vi "M100Utilization1.vi"() -> ()   [LabVIEW 2012]
uses:
  <vilib>/Utility/NIReport.llb/NI_report.lvclass
  <vilib>/addons/database/Connection.llb/DB Tools Open Connec (Path).vi
  <vilib>/addons/database/Connection.llb/Conn Execute.vi
  <vilib>/addons/database/Recordset.llb/Rec Fetch Recordset Data (R).vi
  <vilib>/addons/database/Recordset.llb/Rec Destroy - Connection.vi
  <vilib>/Utility/NIReport.llb/Append Text Table to Report (wrap).vi
  <vilib>/addons/database/_DB Variant To Data/Database Variant To Data.xnode
  <vilib>/addons/database/NI_Database_API.lvlib
  <vilib>/Utility/NIReport.llb/Excel/NI_Excel.lvclass
  <vilib>/addons/_office/NI_ReportGenerationToolkit.lvlib
  <vilib>/Utility/SMTP/NI_SMTPEmail.lvlib
panel:
  in  "Report Template":path=path "O:/Monitor/Report/M100DailyUtilization1.xls"
  out "error out 2":errorcluster
  in  "Table Control":string[][](table)
  out "error out":errorcluster
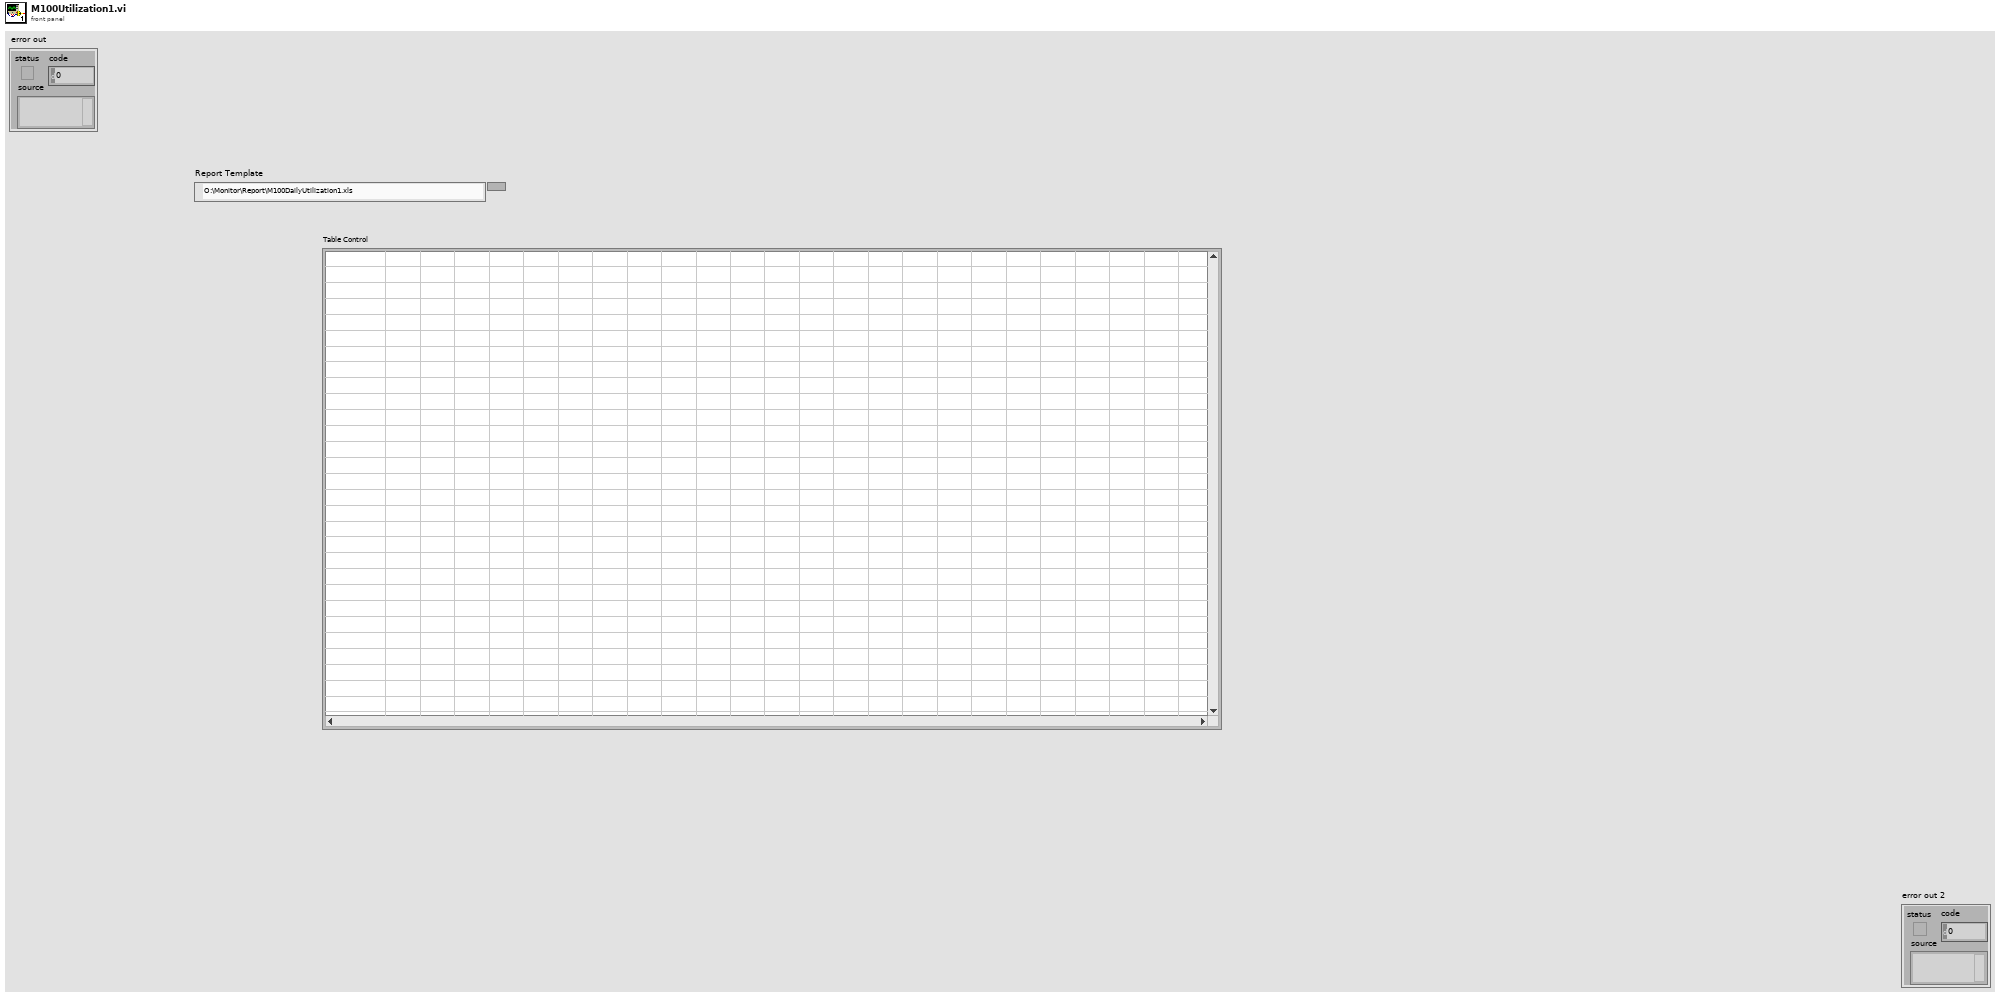
[diagram p1: front panel]
types:
  T1 = typedef "NI_Database_API.lvlib/Conn ObjectReference.ctl" = refnum<k1>
  T2 = typedef "NI_Database_API.lvlib/Rec ObjectReference.ctl" = refnum<k1>
  T3 = enum16{"Standard Report", "HTML", "Word", "Excel"}
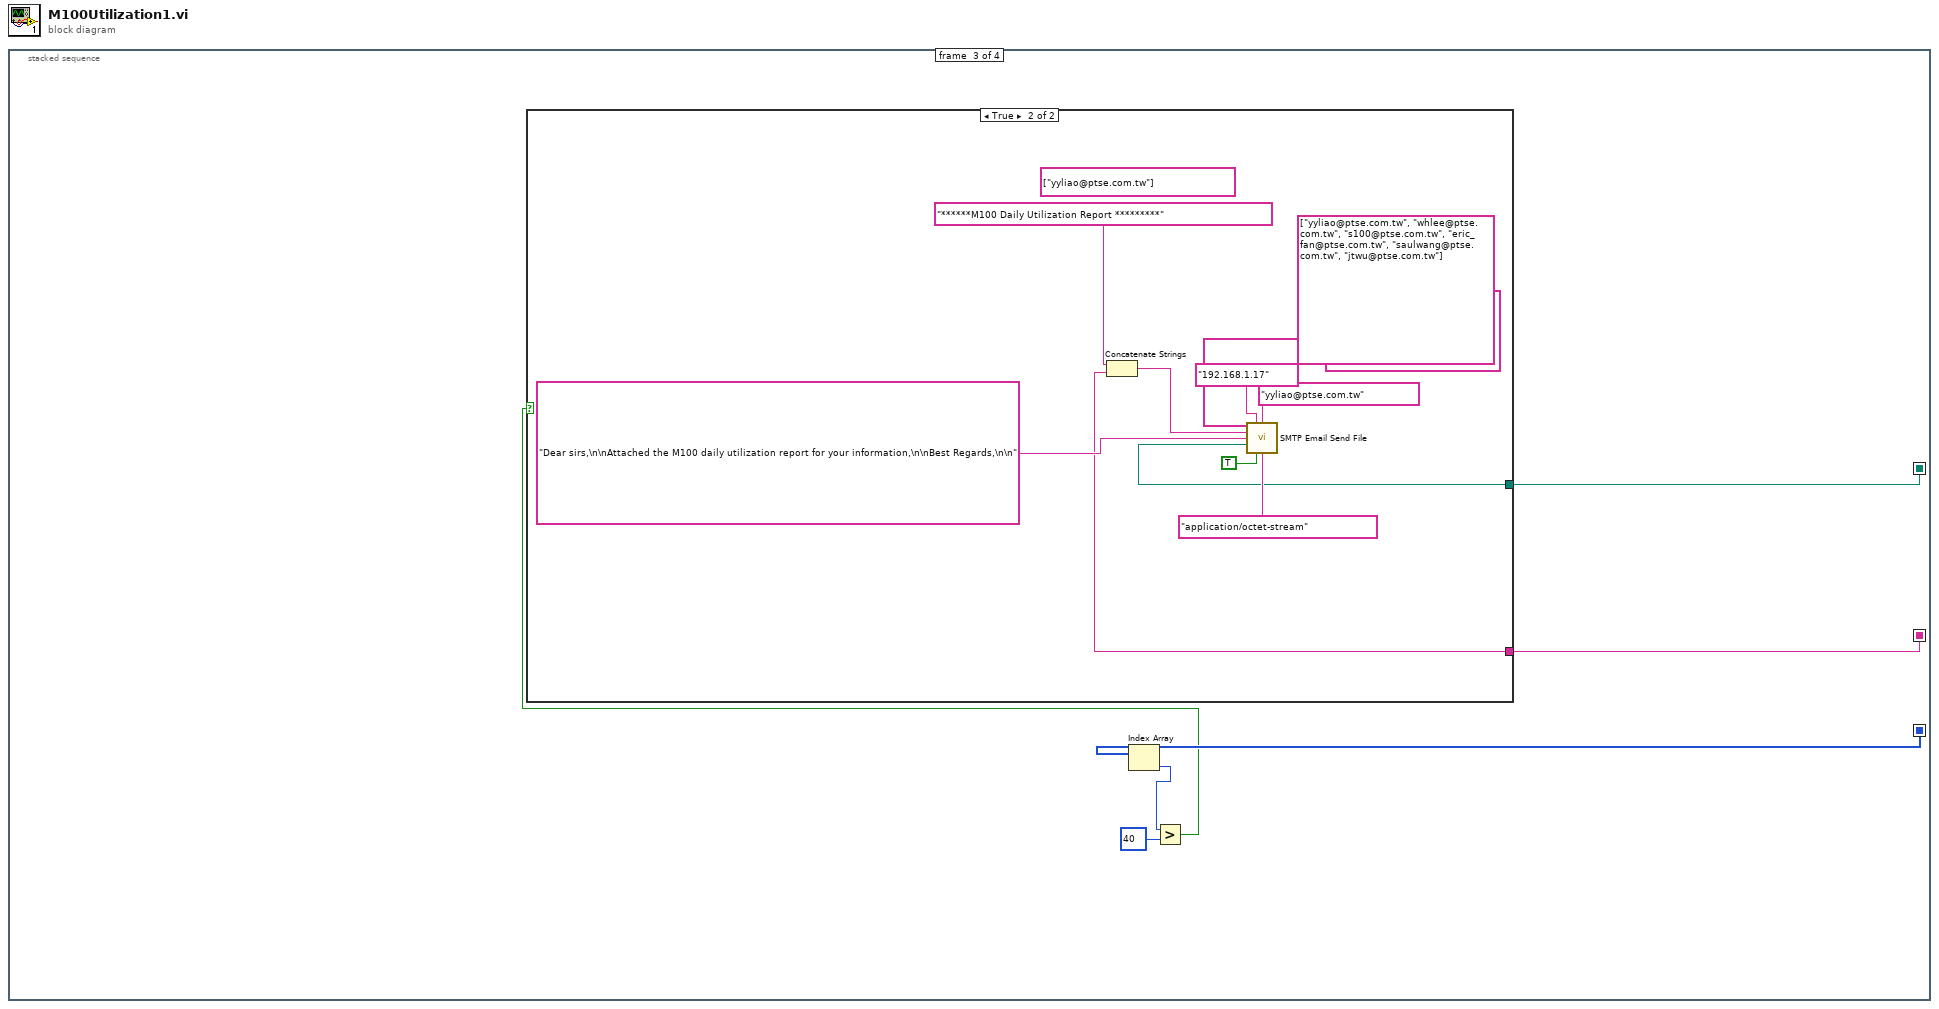
[diagram p0: block diagram]
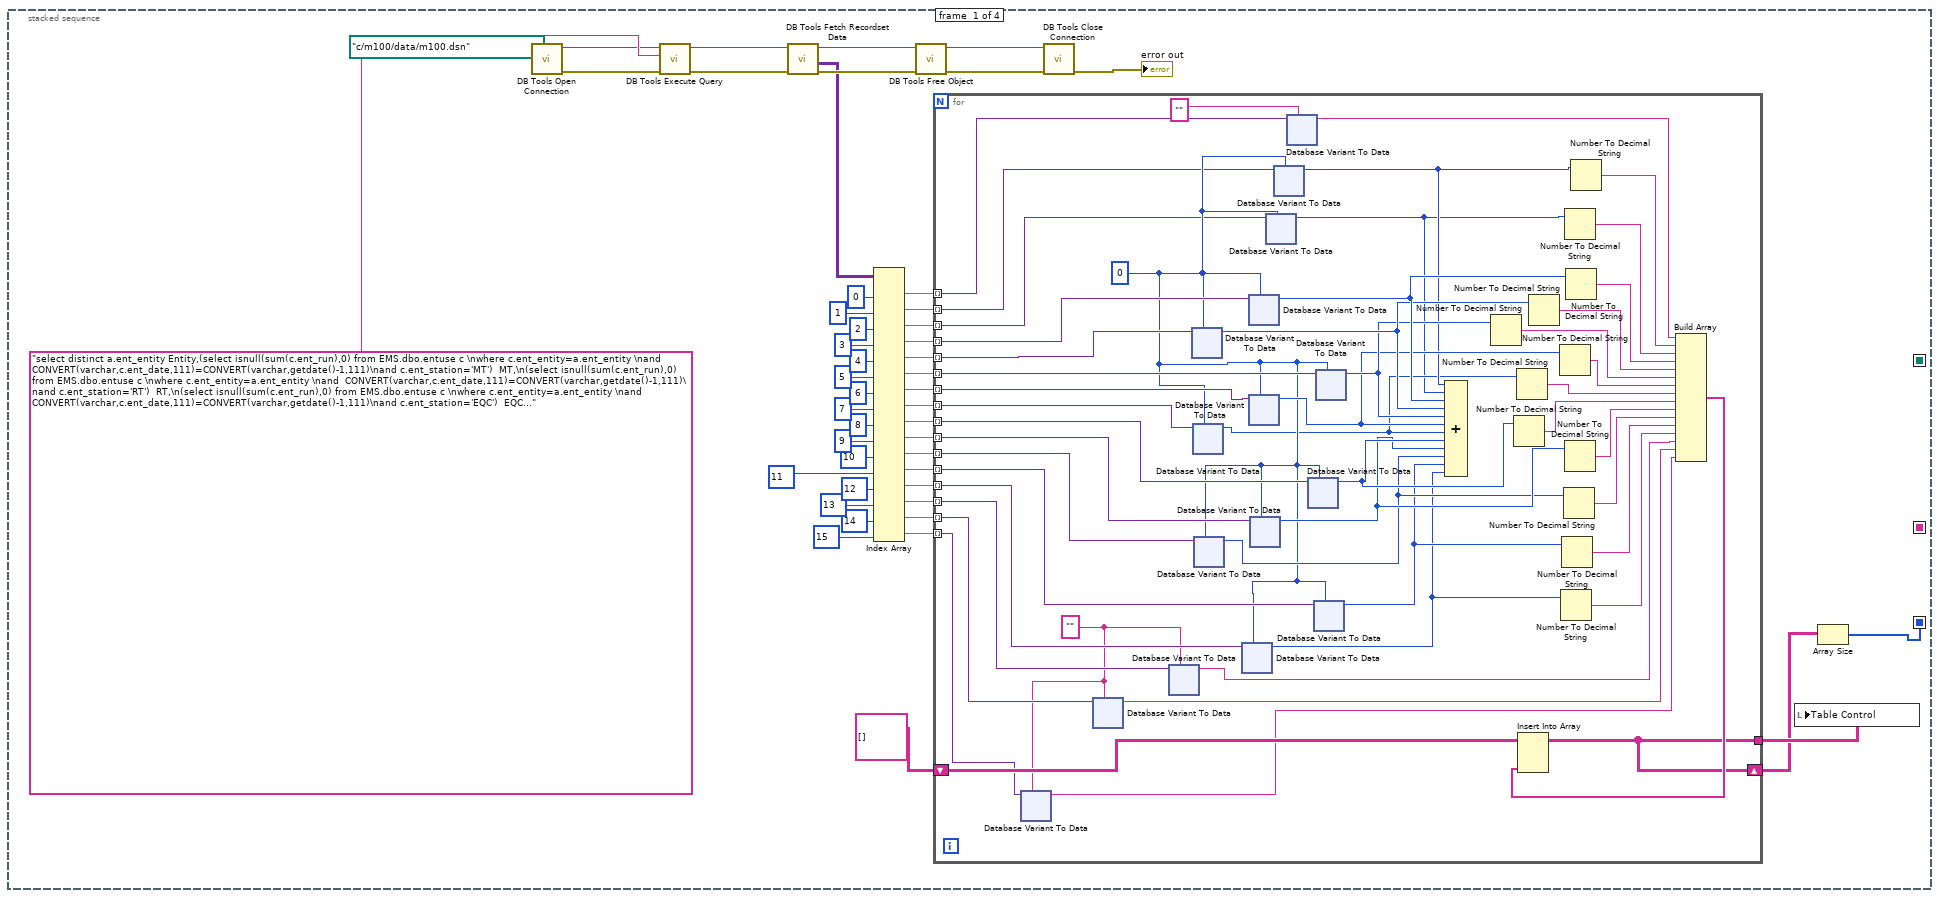
[diagram p2: hidden frame]
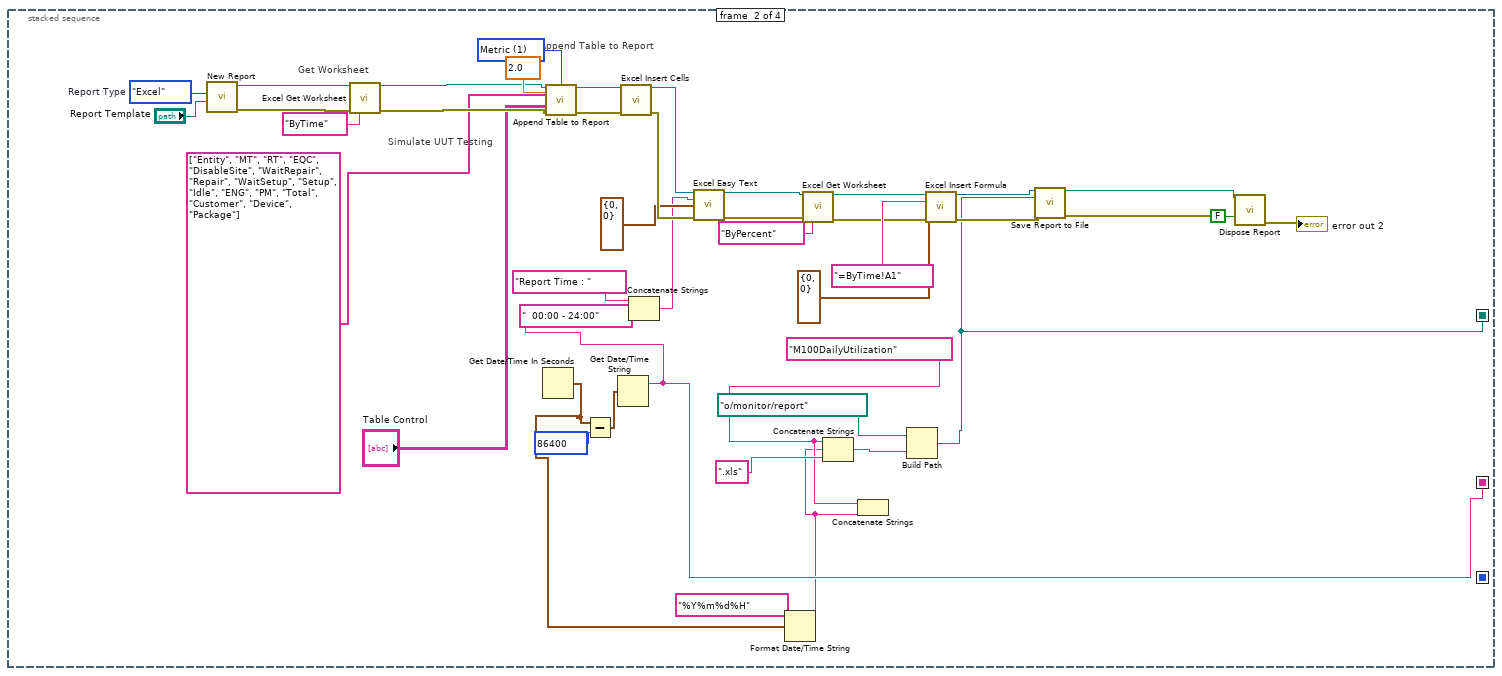
[diagram p3: hidden frame]
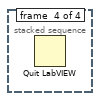
[diagram p5: hidden frame]
diagram:
  n1 = stacked-sequence {
    seq-local: [_ w619 _ _] -> [_ _ w659 _]
    seq-local: [_ w618 _ _] -> [_ _ w658 _]
    seq-local: [w11 _ _ _] -> [_ _ w657 _]
    frame #0 {
      n2 = call-poly <vilib>:"DB Tools Open Connection.vi"("connection information"=path "c:/m100/data/m100.dsn") -> ("error out"=w42:errorcluster, "connection reference"=w46:T1)  [unwired: 7 in]
      n3 = call-poly <vilib>:"DB Tools Execute Query.vi"("error in (no error)"=w42, "SQL query"="select distinct a.ent_entity Entity,(select isnull(sum(c.ent_run),0) from EMS.dbo.entuse c \nwhere c.ent_entity=a.ent_entity \nand  CONVERT(varchar,c.ent_date,111)=CONVERT(varchar,getdate()-1,111)\nand c.ent_station='MT')  MT,\n(select isnull(sum(c.ent_run),0) from EMS.dbo.entuse c \nwhere c.ent_entity=a.ent_entity \nand  CONVERT(varchar,c.ent_date,111)=CONVERT(varchar,getdate()-1,111)\nand c.ent_station='RT')  RT,\n(select isnull(sum(c.ent_run),0) from EMS.dbo.entuse c \nwhere c.ent_entity=a.ent_entity \nand  CONVERT(varchar,c.ent_date,111)=CONVERT(varchar,getdate()-1,111)\nand c.ent_station='EQC')  EQC,sum(ent_runp) OffSite,\nsum(ent_wait_repair) WaitRepair,\n  sum(ent_repair) InRepair,sum(ent_wait_setup) WaitSetup,sum(ent_setup) Setup,\nsum(ent_idle) Idle,sum(ent_eng) Eng,\n  sum(ent_pm) PM,sum(a.ent_time) Total,b.ent_customer,b.ent_product,b.ent_package\nfrom ems.dbo.entuse a,EMS.dbo.ntcent b\n         where CONVERT(varchar,ent_date,111)=CONVERT(varchar,getdate()-1,111)\n              and a.ent_entity not in ('QAMT25','QAMT26','QAMT27','QAMT28')\n and a.ent_entity=b.ent_entity\ngroup by a.ent_entity,b.ent_customer,b.ent_product,b.ent_package\norder by a.ent_entity", "connection reference"=w46) -> ("error out"=w41:errorcluster, "recordset reference"=w45:T2)  [unwired: 5 in]
      n4 = call-poly <vilib>:"DB Tools Fetch Recordset Data.vi"("error in (no error)"=w41, "recordset reference"=w45) -> ("error out"=w40:errorcluster, "recordset data"=w37:variant[][], "recordset reference out"=w44:T2)  [unwired: 3 in]
      n5 = Index Array(array=w37, index (col) #1=0 ("disabled index (col)"), index (col) #2=1 ("index (col)"), index (col) #3=2 ("disabled index (col)"), index (col) #4=3 ("index (col)"), index (col) #5=4 ("index (col)"), index (col) #6=5 ("index (col)"), index (col) #7=6 ("index (col)"), index (col) #8=7 ("index (col)"), index (col) #9=8 ("index (col)"), index (col) #10=9 ("index (col)"), index (col) #11=10 ("index (col)"), index (col) #12=11 ("index (col)"), index (col) #13=12 ("index (col)"), index (col) #14=13 ("index (col)"), index (col) #15=14 ("index (col)"), index (col) #16=15 ("index (col)")) -> (element #1=w2:variant[], element #2=w1:variant[], element #3=w25:variant[], element #4=w24:variant[], element #5=w23:variant[], element #6=w22:variant[], element #7=w21:variant[], element #8=w20:variant[], element #9=w19:variant[], element #10=w18:variant[], element #11=w17:variant[], element #12=w16:variant[], element #13=w15:variant[], element #14=w8:variant[], element #15=w7:variant[], element #16=w5:variant[])  [unwired: 16 in]
      n6 = call-poly <vilib>:"DB Tools Free Object.vi"("error in (no error)"=w40, "recordset reference"=w44) -> ("error out"=w39:errorcluster, "connection reference"=w43:T1)  [unwired: 8 in]
      n7 = for {
        tunnel: w25 -> [w54] mode=indexing
        tunnel: w24 -> [w98] mode=indexing
        tunnel: w23 -> [w97] mode=indexing
        tunnel: w22 -> [w96] mode=indexing
        tunnel: w21 -> [w95] mode=indexing
        tunnel: w20 -> [w94] mode=indexing
        tunnel: w19 -> [w93] mode=indexing
        tunnel: w18 -> [w92] mode=indexing
        tunnel: w17 -> [w91] mode=indexing
        tunnel: w16 -> [w90] mode=indexing
        tunnel: w15 -> [w89] mode=indexing
        tunnel: [w67] -> w13
        shift-right: [w67] -> w12
        shift-left: string[][] [] ("array") -> [w66]
        tunnel: w8 -> [w65] mode=indexing
        tunnel: w7 -> [w64] mode=indexing
        tunnel: w5 -> [w61] mode=indexing
        tunnel: w2 -> [w57] mode=indexing
        tunnel: w1 -> [w55] mode=indexing
        w60 = ""
        w56 = 0
        n8 = xnode "Database Variant To Data"("database variant"=w61, "type"=w60) -> ("data"=w59:string)  [unwired: 1 in, 1 out]
        n9 = xnode "Database Variant To Data"("database variant"=w64, "type"=w60) -> ("data"=w62:string)  [unwired: 1 in, 1 out]
        n10 = xnode "Database Variant To Data"("database variant"=w65, "type"=w60) -> ("data"=w63:string)  [unwired: 1 in, 1 out]
        n11 = xnode "Database Variant To Data"("database variant"=w97, "type"=w56) -> ("data"=w85:i32)  [unwired: 1 in, 1 out]
        n12 = xnode "Database Variant To Data"("database variant"=w94, "type"=w56) -> ("data"=w50:i32)  [unwired: 1 in, 1 out]
        n13 = xnode "Database Variant To Data"("database variant"=w91, "type"=w56) -> ("data"=w74:i32)  [unwired: 1 in, 1 out]
        n14 = xnode "Database Variant To Data"("database variant"=w89, "type"=w56) -> ("data"=w70:i32)  [unwired: 1 in, 1 out]
        n15 = xnode "Database Variant To Data"("database variant"=w98, "type"=w56) -> ("data"=w87:i32)  [unwired: 1 in, 1 out]
        n16 = xnode "Database Variant To Data"("database variant"=w95, "type"=w56) -> ("data"=w81:i32)  [unwired: 1 in, 1 out]
        n17 = xnode "Database Variant To Data"("database variant"=w92, "type"=w56) -> ("data"=w76:i32)  [unwired: 1 in, 1 out]
        n18 = xnode "Database Variant To Data"("database variant"=w54, "type"=w56) -> ("data"=w49:i32)  [unwired: 1 in, 1 out]
        n19 = xnode "Database Variant To Data"("database variant"=w55, "type"=w56) -> ("data"=w51:i32)  [unwired: 1 in, 1 out]
        n20 = xnode "Database Variant To Data"("database variant"=w57, "type"="") -> ("data"=w58:string)  [unwired: 1 in, 1 out]
        n21 = xnode "Database Variant To Data"("database variant"=w93, "type"=w56) -> ("data"=w78:i32)  [unwired: 1 in, 1 out]
        n22 = xnode "Database Variant To Data"("database variant"=w90, "type"=w56) -> ("data"=w72:i32)  [unwired: 1 in, 1 out]
        n23 = xnode "Database Variant To Data"("database variant"=w96, "type"=w56) -> ("data"=w83:i32)  [unwired: 1 in, 1 out]
        n24 = Compound Arithmetic op=ADD(w51, w49, w87, w85, w83, w81, w50, w78, w76, w74, w72, w70) -> ()  [unwired: 1 out]
        n25 = Number To Decimal String(number=w83) -> (decimal integer string=w82:string)  [unwired: 1 in]
        n26 = Number To Decimal String(number=w78) -> (decimal integer string=w77:string)  [unwired: 1 in]
        n27 = Number To Decimal String(number=w50) -> (decimal integer string=w79:string)  [unwired: 1 in]
        n28 = Number To Decimal String(number=w85) -> (decimal integer string=w84:string)  [unwired: 1 in]
        n29 = Number To Decimal String(number=w81) -> (decimal integer string=w80:string)  [unwired: 1 in]
        n30 = Number To Decimal String(number=w70) -> (decimal integer string=w69:string)  [unwired: 1 in]
        n31 = Number To Decimal String(number=w72) -> (decimal integer string=w71:string)  [unwired: 1 in]
        n32 = Number To Decimal String(number=w74) -> (decimal integer string=w73:string)  [unwired: 1 in]
        n33 = Number To Decimal String(number=w49) -> (decimal integer string=w52:string)  [unwired: 1 in]
        n34 = Number To Decimal String(number=w76) -> (decimal integer string=w75:string)  [unwired: 1 in]
        n35 = Number To Decimal String(number=w87) -> (decimal integer string=w86:string)  [unwired: 1 in]
        n36 = Number To Decimal String(number=w51) -> (decimal integer string=w53:string)  [unwired: 1 in]
        n37 = Build Array(w58, w53, w52, w86, w84, w82, w80, w79, w77, w75, w73, w71, w69, w63, w62, w59) -> (w68:string[])
        n38 = Insert Into Array(array=w66, new element=w68) -> (w67:string[][])  [unwired: 2 in]
      }
      n39 = call <vilib>:"DB Tools Close Connection.vi"("error in (no error)"=w39, "connection reference"=w43) -> ("error out"=→"error out":errorcluster)  [unwired: 5 in]
      n40 = local write "Table Control"(w13) -> ()
      n41 = Array Size(array=w12) -> (size(s)=w11:i32[])
    }
    frame #1 {
      w615 = u16 1 items=["US", "Metric", "Default"] ("measurement system")
      w620 = "M100DailyUtilization"
      w653 = T3."Excel"  # Report Type
      # "Simulate UUT Testing"
      # "Append Table to Report"
      # "Get Worksheet"
      n42 = call <vilib>:"New Report.vi"("report type"=w653, "template (empty)"="Report Template") -> ("report out"=w648:refnum<class "NI_report.lvclass">, "error out"=w647:errorcluster)  [unwired: 12 in]
      n43 = call <vilib>:"Excel Get Worksheet.vi"("report in"=w648, "error in (no error)"=w647, "name (\"\")"="ByTime" ("name (\"\")")) -> ("report out"=w637:refnum<class "NI_report.lvclass">, "error out"=w636:errorcluster)  [unwired: 11 in]
      n44 = Get Date/Time In Seconds() -> (seconds since 1Jan1904=w612:timestamp)
      n45 = call-poly <vilib>:"Append Table to Report.vi"("report in"=w637, "column width (1)"=2.0, "measurement system"=w615, "column headers"=string[] ["Entity", "MT", "RT", "EQC", "DisableSite", "WaitRepair", "Repair", "WaitSetup", "Setup", "Idle", "ENG", "PM", "Total", "Customer", "Device", "Package"] ("row headers"), "text data"="Table Control", "error in (no error)"=w636) -> ("report out"=w650:refnum<class "NI_report.lvclass">, "error out"=w649:errorcluster)  [unwired: 6 in, 2 out]
      n46 = Subtract(x=w612, y=86400) -> (x-y=w616:timestamp)
      n47 = Get Date/Time String(seconds (now)=w616) -> (date string=w618:string)  [unwired: 2 in, 1 out]
      n48 = call <vilib>:"Excel Insert Cells.vi"("report in"=w650, "error in (no error)"=w649) -> ("report out"=w644:refnum<class "NI_report.lvclass">, "error out"=w643:errorcluster)  [unwired: 12 in]
      n49 = Concatenate Strings("Report Time : " ("string"), w618, "  00:00 - 24:00" ("string")) -> (w640:string)
      n50 = call <vilib>:"Excel Easy Text.vi"("report in"=w644, "text"=w640, "start (-1, -1)"=cluster{"row":i32, "column":i32} {"row"=0, "column"=0} ("end (-1, -1)"), "error in (no error)"=w643) -> ("report out"=w632:refnum<class "NI_report.lvclass">, "error out"=w631:errorcluster)  [unwired: 7 in, 3 out]
      n51 = Format Date/Time String(time format string (%c)="%Y%m%d%H", seconds (now)=w612) -> (date/time string=w613:string)  [unwired: 1 in]
      n52 = call <vilib>:"Excel Get Worksheet.vi"("report in"=w632, "error in (no error)"=w631, "name (\"\")"="ByPercent" ("name (\"\")")) -> ("report out"=w627:refnum<class "NI_report.lvclass">, "error out"=w626:errorcluster)  [unwired: 11 in]
      n53 = Concatenate Strings(w620, w613, ".xls" ("string")) -> (w621:string)
      n54 = Concatenate Strings(w620, w613) -> ()  [unwired: 1 out]
      n55 = Build Path(base path=path "o:/monitor/report", name or relative path=w621) -> (appended path=w619:path)
      n56 = call <vilib>:"Excel Insert Formula.vi"("report in"=w627, "formula"="=ByTime!A1", "start (0, 0)"=cluster{"row":i32, "column":i32} {"row"=0, "column"=0}, "error in (no error)"=w626) -> ("report out"=w625:refnum<class "NI_report.lvclass">, "error out"=w624:errorcluster)  [unwired: 10 in]
      n57 = call-dynamic "Save Report to File.vi"("report in"=w625, "report file path"=w619, "error in (no error)"=w624) -> ("report out"=w639:refnum<class "NI_report.lvclass">, "error out"=w638:errorcluster)  [unwired: 11 in]
      n58 = call-dynamic "Dispose Report.vi"("report in"=w639, "save changes? (F)"=FALSE, "error in (no error)"=w638) -> ("error out"=→"error out 2":errorcluster)  [unwired: 12 in]
    }
    frame #2 {
      n59 = Index Array(array=w657) -> (element=w656:i32)  [unwired: 1 in]
      n60 = Greater?(x=w656, y=40) -> (0:w654:bool)
      n61 = case shown="True" w654 {
        tunnel: w659 -> [_ w664]
        tunnel: w658 -> [_ w662]
        frame False {
        }
        frame True {
          (unwired) string[] ["yyliao@ptse.com.tw"] ("recipients")
          n62 = Concatenate Strings("******M100 Daily Utilization Report *********" ("subject ([No Subject])"), w662) -> (w661:string)
          n63 = call <vilib>:"SMTP Email Send File.vi"("recipients"=string[] ["yyliao@ptse.com.tw", "whlee@ptse.com.tw", "s100@ptse.com.tw", "eric_fan@ptse.com.tw", "saulwang@ptse.com.tw", "jtwu@ptse.com.tw"], "mail server"="192.168.1.17", "return address"="yyliao@ptse.com.tw", "subject ([No Subject])"=w661, "message"="Dear sirs,\n\nAttached the M100 daily utilization report for your information,\n\nBest Regards,\n\n", "file path"=w664, "binary? (F)"=TRUE, "MIME content-type (application/octet-stream)"="application/octet-stream") -> ()  [unwired: 6 in, 2 out]
        }
      }
    }
    frame #3 {
      n64 = Quit LabVIEW() -> ()  [unwired: 1 in]
    }
  }
